vi "create_data_folder.vi"(8 "error in (no error)":errorcluster, 11 "ExperimentVariables in":refnum<class "ExperimentVariables.lvclass">) -> (0 "error out":errorcluster, 3 "ExperimentVariables out":refnum<class "ExperimentVariables.lvclass">)   [LabVIEW 2012, in "ExperimentVariables.lvclass"]
uses:
  ExperimentVariables.lvclass
  ExperimentVariables.lvclass/ExperimentVariables.ctl
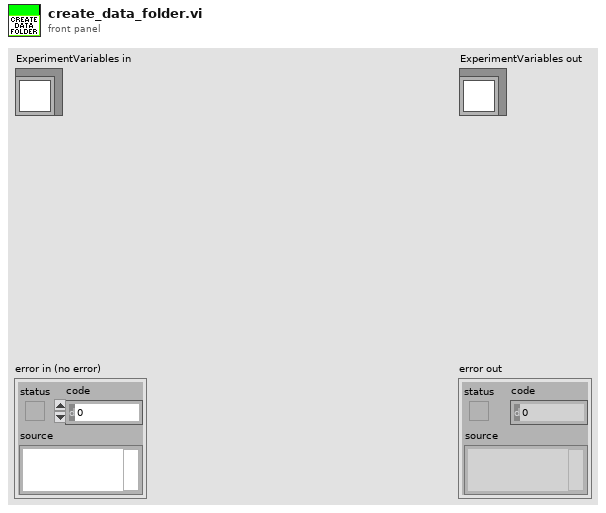
[diagram p1: front panel]
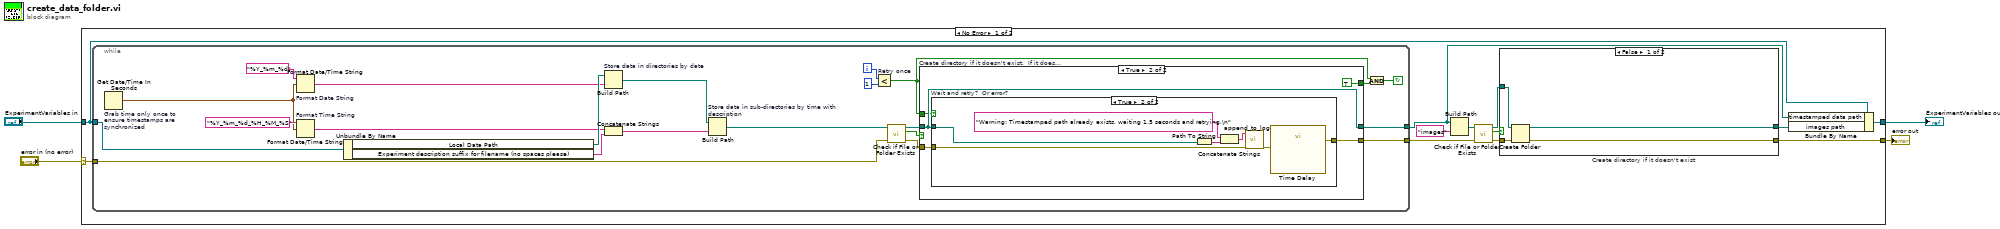
[diagram p0: block diagram]
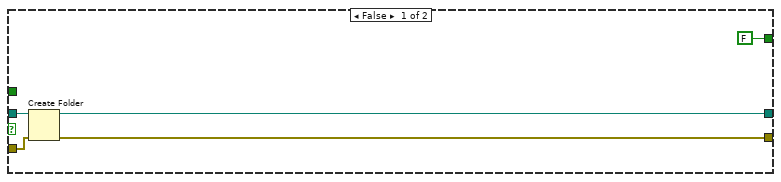
[diagram p2: hidden frame]
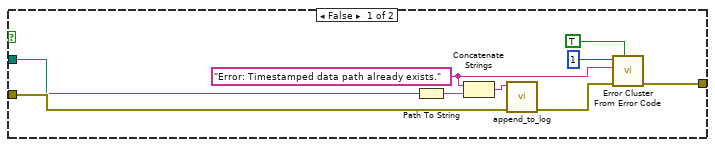
[diagram p3: hidden frame]
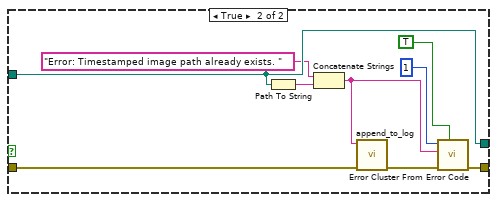
[diagram p4: hidden frame]
diagram:
  n1 = case shown="No Error" "error in (no error)" {
    selector: "error in (no error)" -> [w8 w79]
    tunnel: [w10 w79] -> w3
    tunnel: [w16 w78] -> w1
    tunnel: "ExperimentVariables in" -> [w6 w78]
    frame No Error {
      n2 = while {
        tunnel: w8 -> [w24]
        tunnel: [w23] -> w7
        tunnel: [w22] -> w5
        tunnel: w6 -> [w21]
        i -> [w38]
        stop <- w20 continue-if-true
        n3 = Get Date/Time In Seconds "Grab time only once to ensure timestamps are synchronized"() -> (seconds since 1Jan1904=w17:timestamp)
        n4 = Format Date/Time String "Format Date String"(time format string (%c)="%Y_%m_%d", seconds (now)=w17) -> (date/time string=w25:string)  [unwired: 1 in]
        n5 = Format Date/Time String "Format Time String"(time format string (%c)="%Y_%m_%d_%H_%M_%S", seconds (now)=w17) -> (date/time string=w32:string)  [unwired: 1 in]
        n6 = Unbundle By Name(w21) -> ("Local Data Path"=w34:path, "Experiment description suffix for filename (no spaces please)"=w35:string)
        n7 = Build Path "Store data in directories by date"(base path=w34, name or relative path=w25) -> (appended path=w31:path)
        n8 = Concatenate Strings(w32, w35) -> (w33:string)
        n9 = Build Path "Store data in sub-directories by time with description"(base path=w31, name or relative path=w33) -> (appended path=w36:path)
        n10 = Less? "Retry once"(x=w38, y=1) -> (x < y?=w18:bool)
        n11 = call <vilib>:"Check if File or Folder Exists.vi"("error in (no error)"=w24, "path"=w36) -> ("error out"=w27:errorcluster, "file or folder exists?"=w28:bool, "dup path"=w29:path)  [unwired: 7 in]
        n12 = case "Create directory if it doesn't exist.  If it does..." shown="True" w28 {
          tunnel: w27 -> [w43 w47]
          tunnel: [w42 w46] -> w23
          tunnel: w29 -> [w40 w48]
          tunnel: [w41 w48] -> w22
          tunnel: w18 -> [_ w45]
          tunnel: [FALSE TRUE] -> w19
          frame False {
            n13 = Create Folder(path (use dialog)=w40, error in=w43) -> (created path=w41:path, error out=w42:errorcluster)  [unwired: 1 in, 1 out]
          }
          frame True {
            n14 = case "Wait and retry?  Or error?" shown="True" w45 {
              tunnel: w48 -> [w55 w64]
              tunnel: w47 -> [w56 w61]
              tunnel: [w53 w59] -> w46
              frame False {
                w51 = "Error: Timestamped data path already exists." ("string")
                n15 = Path To String(path=w55) -> (string=w57:string)
                n16 = Concatenate Strings(w51, w57) -> (w52:string)
                n17 = call "append_to_log.vi"("error in"=w56, "string"=w52) -> ("error out"=w54:errorcluster)  [unwired: 9 in]
                n18 = call <vilib>:"Error Cluster From Error Code.vi"("show call chain? (False)"=TRUE, "error in (no error)"=w54, "error message (\"\")"=w51, "error code (0)"=1) -> ("error out"=w53:errorcluster)  [unwired: 5 in]
              }
              frame True {
                n19 = Path To String(path=w64) -> (string=w63:string)
                n20 = Concatenate Strings("Warning: Timestamped path already exists, waiting 1.5 seconds and retrying.\n" ("string"), w63) -> (w58:string)
                n21 = call "append_to_log.vi"("error in"=w61, "string"=w58) -> ("error out"=w60:errorcluster)  [unwired: 9 in]
                n22 = call "Time Delay"("error in (no error)"=w60) -> ("error out"=w59:errorcluster)  [unwired: 10 in]
              }
            }
          }
        }
        n23 = And(x=w18, y=w19) -> (x .and. y?=w20:bool)
      }
      n24 = Build Path(base path=w5, name or relative path="images") -> (appended path=w14:path)
      n25 = call <vilib>:"Check if File or Folder Exists.vi"("error in (no error)"=w7, "path"=w14) -> ("error out"=w13:errorcluster, "file or folder exists?"=w12:bool, "dup path"=w11:path)  [unwired: 7 in]
      n26 = case "Create directory if it doesn't exist" shown="False" w12 {
        tunnel: w13 -> [w68 w74]
        tunnel: [w67 w72] -> w10
        tunnel: w11 -> [w65 w77]
        tunnel: [w66 w77] -> w9
        frame False {
          n27 = Create Folder(path (use dialog)=w65, error in=w68) -> (created path=w66:path, error out=w67:errorcluster)  [unwired: 1 in, 1 out]
        }
        frame True {
          n28 = Path To String(path=w77) -> (string=w76:string)
          n29 = Concatenate Strings("Error: Timestamped image path already exists. " ("string"), w76) -> (w70:string)
          n30 = call "append_to_log.vi"("error in"=w74, "string"=w70) -> ("error out"=w73:errorcluster)  [unwired: 9 in]
          n31 = call <vilib>:"Error Cluster From Error Code.vi"("show call chain? (False)"=TRUE, "error in (no error)"=w73, "error message (\"\")"=w70, "error code (0)"=1) -> ("error out"=w72:errorcluster)  [unwired: 5 in]
        }
      }
      n32 = Bundle By Name(cluster=w6, "timestamped data path"=w5, "images path"=w9) -> (w16:refnum<class "ExperimentVariables.lvclass">)
    }
    frame Error {
    }
  }
  "error out" <- w3
  "ExperimentVariables out" <- w1
